vi "getPos.vi"(8 "error in (no error)":errorcluster caption="错误输入（无错误）", 10 "lab or motor":enum16{"lab", "motor"}(ring), 11 "OneMotion 输入":refnum<class "OneMotion.lvclass">) -> (0 "error out":errorcluster caption="错误输出", 2 "pos":dbl, 3 "OneMotion 输出":refnum<class "OneMotion.lvclass">)   [LabVIEW 2016, in "MotionControl_UFO_3DOF.lvlib" / "OneMotion.lvclass"]
uses:
  <userlib>/MotionControl_UFO_3DOF/OneMotion/OneMotion.lvclass
  <userlib>/MotionControl_UFO_3DOF/OneMotion/OneMotion.lvclass/OneMotion.ctl
  <userlib>/MotionControl_UFO_3DOF/StepMotor/StepMotor.lvclass
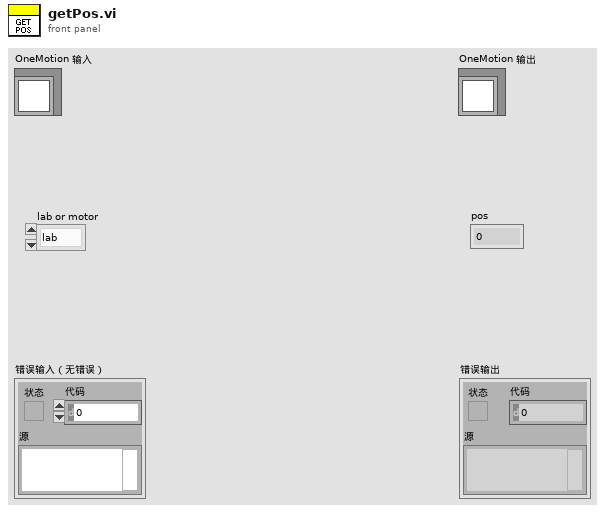
[diagram p1: front panel]
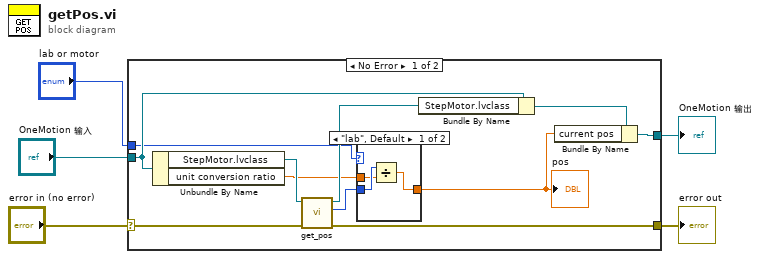
[diagram p0: block diagram]
diagram:
  n1 = case shown="No Error" "error in (no error)" {
    selector: "error in (no error)" -> [w13 w22]
    tunnel: [w6 w22] -> w4
    tunnel: [w9 w21] -> w2
    tunnel: "OneMotion 输入" -> [w15 w21]
    tunnel: "lab or motor" -> [w12 _]
    frame No Error {
      n2 = Unbundle By Name(w15) -> ("StepMotor.lvclass"=w16:refnum<class "StepMotor.lvclass">, "unit conversion ratio"=w8:dbl)
      n3 = call-dynamic "get_pos.vi"("error in (no error)"=w13, "StepMotor 输入"=w16) -> ("error out"=w6:errorcluster, "pos"=w11:i32, "StepMotor 输出"=w14:refnum<class "StepMotor.lvclass">)  [unwired: 7 in]
      n4 = case shown="\"lab\", Default" w12 {
        tunnel: w11 -> [w18 w20]
        tunnel: [w19 w20] -> w10
        tunnel: w8 -> [w17 _]
        frame "lab", Default {
          n5 = Divide(x=w18, y=w17) -> (x/y=w19:dbl)
        }
        frame "motor" {
        }
      }
      "pos" <- w10
      n6 = Bundle By Name(cluster=w15, "StepMotor.lvclass"=w14) -> (w7:refnum<class "OneMotion.lvclass">)
      n7 = Bundle By Name(cluster=w7, "current pos"=w10) -> (w9:refnum<class "OneMotion.lvclass">)
    }
    frame Error {
    }
  }
  "error out" <- w4
  "OneMotion 输出" <- w2
